vi "BuildDIrectoryTree.vi"(2 "CallingVI":refnum<vi>, 3 "Tree Refnum":refnum<vi>, 4 "Folder Path":path) -> ()   [LabVIEW 2014]
panel:
  out "folder tags":string[](array[string])
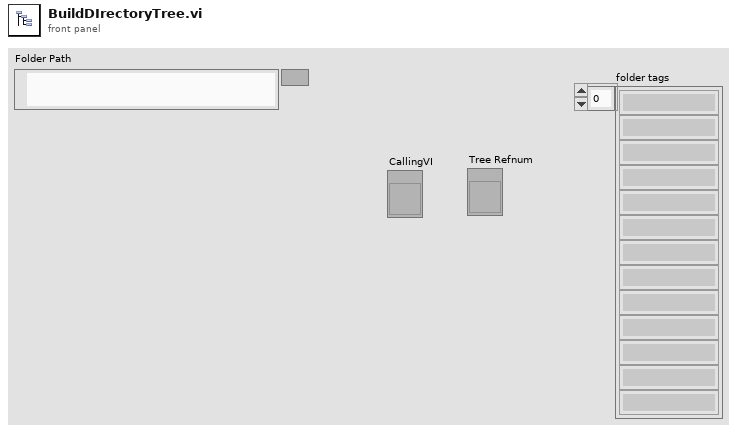
[diagram p1: front panel]
types:
  T1 = cluster{"name":string, i32, "name":string, string[]}[]
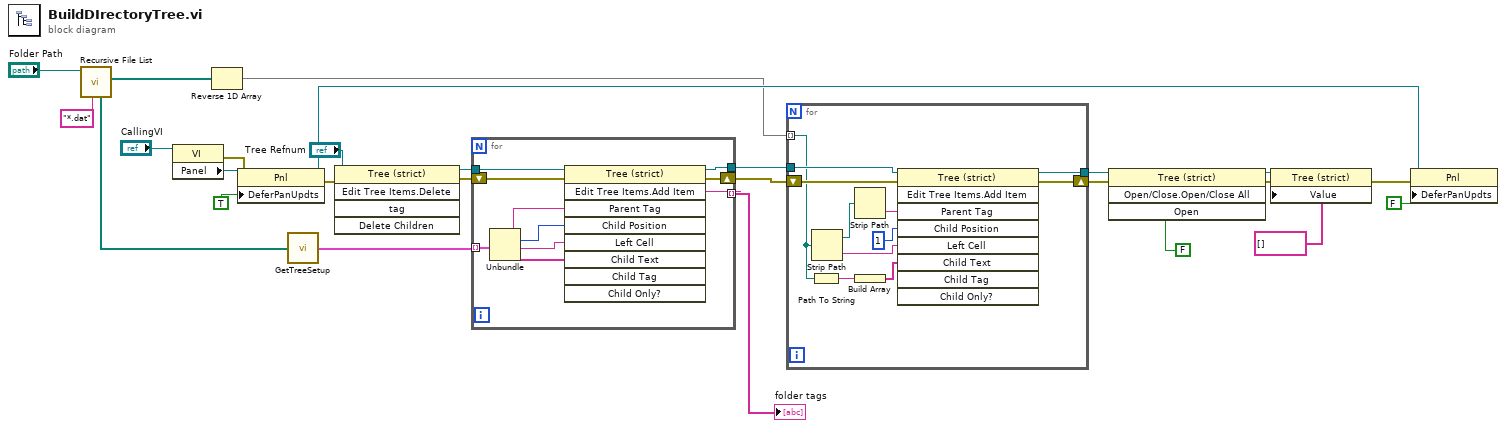
[diagram p0: block diagram]
diagram:
  n1 = call <vilib>:"Recursive File List.vi"("pattern"="*.dat", "Folder Path"="Folder Path") -> ("All Files in Dir"=w19:path[], "All Folders"=w6:path[])  [unwired: 5 in, 3 out]
  n2 = property class="VI"(reference="CallingVI") -> (error out=w15:errorcluster, "Panel"=w18:refnum<vi>)  [unwired: 1 in, 1 out]
  n3 = Reverse 1D Array(array=w19) -> (reversed array=w7:path[])
  n4 = property class="Pnl"(reference=w18, error in=w15, "DeferPanUpdts"=TRUE ("Defer Panel Updates")) -> (reference out=w14:refnum<vi>, error out=w1:errorcluster)
  n5 = call "GetTreeSetup.vi"("All Folders"=w6) -> ("Format"=w3:T1)
  n6 = invoke on="Invoke Node" class="Tree (strict)" method="Edit Tree Items.Delete"(reference="Tree Refnum", error in=w1) -> (reference out=w22:refnum<vi>, error out=w26:errorcluster)  [unwired: 3 in, 3 out]
  n7 = for {
    shift-right: [w35] -> w25
    shift-left: w26 -> [w36]
    tunnel: w22 -> [w34]
    tunnel: [w33] -> w21
    tunnel: [w32] -> w8 mode=indexing
    tunnel: w3 -> [w31] mode=indexing
    # "Populate the tree items"
    n8 = Unbundle(w31) -> ("name"=w30:string, w29:i32, "name"=w28:string, w27:string[])
    n9 = invoke on="Invoke Node" class="Tree (strict)" method="Edit Tree Items.Add Item"(reference=w34, error in=w36, "Parent Tag"=w30, "Child Position"=w29, "Left Cell"=w28, "Child Text"=w27) -> (reference out=w33:refnum<vi>, error out=w35:errorcluster, "Edit Tree Items:Add Item"=w32:string)  [unwired: 3 in, 6 out]
  }
  "folder tags" <- w8
  n10 = for {
    tunnel: w7 -> [w37] mode=indexing
    shift-right: [w46] -> w24
    shift-left: w25 -> [w47]
    tunnel: w21 -> [w45]
    tunnel: [w44] -> w20
    n11 = Path To String(path=w37) -> (string=w39:string)
    n12 = Strip Path(path=w37) -> (stripped path=w43:path, name=w41:string)
    n13 = Strip Path(path=w43) -> (name=w42:string)  [unwired: 1 out]
    n14 = Build Array(w39) -> (w38:string[])
    n15 = invoke on="Invoke Node" class="Tree (strict)" method="Edit Tree Items.Add Item"(reference=w45, error in=w47, "Parent Tag"=w42, "Child Position"=1, "Left Cell"=w41, "Child Text"=w38) -> (reference out=w44:refnum<vi>, error out=w46:errorcluster)  [unwired: 3 in, 7 out]
  }
  n16 = invoke on="Invoke Node" class="Tree (strict)" method="Open/Close.Open/Close All"(reference=w20, error in=w24, "Open"=FALSE ("Open?")) -> (reference out=w12:refnum<vi>, error out=w11:errorcluster)  [unwired: 1 in, 2 out]
  n17 = property class="Tree (strict)"(reference=w12, error in=w11, "Value"=string[] []) -> (error out=w10:errorcluster)  [unwired: 1 out]
  n18 = property class="Pnl"(reference=w14, error in=w10, "DeferPanUpdts"=FALSE ("Defer Panel Updates")) -> ()  [unwired: 2 out]
